vi "Generate z stage position array.vi"(8 "Error In":errorcluster, 11 "X Axis":T1) -> (0 "Error Out":errorcluster, 3 "X Scale":dbl[](array[numeric]))   [LabVIEW 2018]
uses:
  <vilib>/Analysis/1siggen.llb/Ramp Pattern by Samples.vi
  <vilib>/Analysis/NI_AALBase.lvlib
panel:
  out "Ramp Pattern":dbl[](array[numeric])
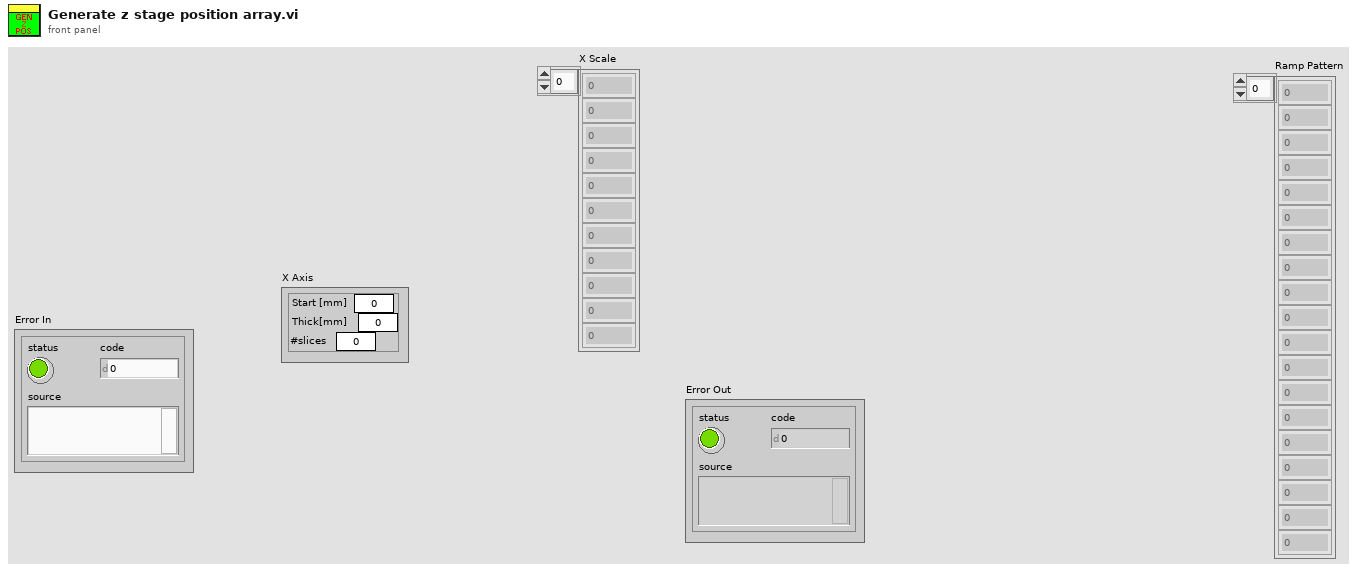
[diagram p1: front panel]
types:
  T1 = cluster{"Start [mm]":dbl, "Thick[mm]":dbl, "#slices":u16}
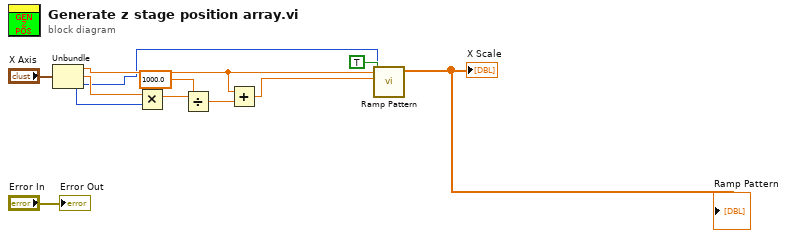
[diagram p0: block diagram]
diagram:
  n1 = Unbundle("X Axis") -> ("Start [mm]"=w4:dbl, "Thick[mm]"=w8:dbl, "#slices"=w1:u16)
  n2 = Multiply(x=w8, y=w1) -> (x*y=w7:dbl)
  n3 = Divide(x=w7, y=1000.0) -> (x/y=w5:dbl)
  n4 = Add(x=w4, y=w5) -> (x+y=w3:dbl)
  n5 = call-poly <vilib>:"Ramp Pattern.vi"("exclude end?"=TRUE, "start"=w4, "end"=w3, "samples"=w1) -> ("Ramp Pattern"=→"X Scale" →"Ramp Pattern":dbl[])  [unwired: 6 in, 1 out]
  "Error Out" <- "Error In"
